vi "Construct.vi"(8 "error in (no error)":errorcluster, 11 "reference in":refnum<class "BrowerGuidencer.lvclass">) -> (0 "error out":errorcluster, 2 "BrowerComponent":refnum<class "BrowerComponent.lvclass">, 3 "reference out":refnum<class "BrowerGuidencer.lvclass">)   [LabVIEW 2015, in "BrowerGuidencer.lvclass"]
uses:
  BrowerGuidencer.lvclass
  BrowerComponent/BrowerComponent/BrowerComponent.lvclass
  BrowerGuidencer.lvclass/BrowerGuidencer.ctl
  AbstractBuilder/AbstractBuilder.lvclass
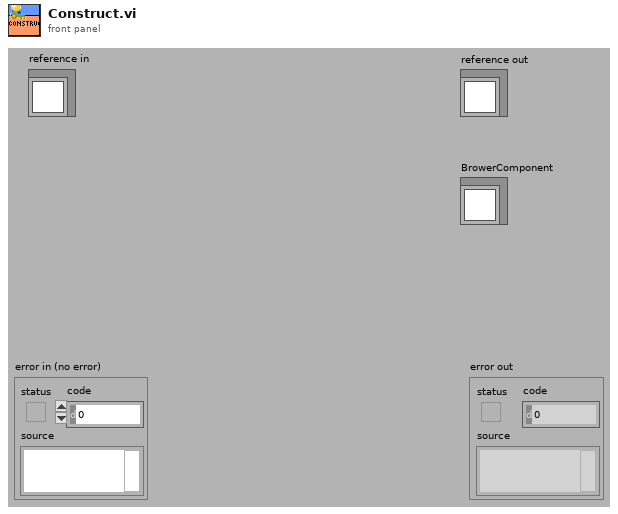
[diagram p1: front panel]
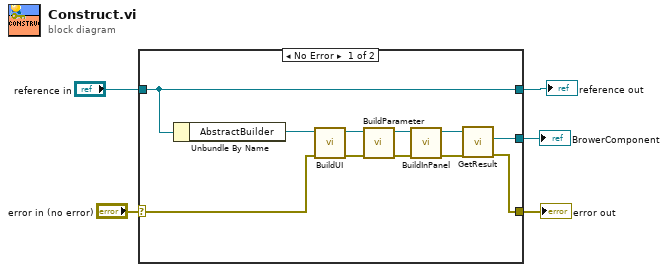
[diagram p0: block diagram]
diagram:
  n1 = case shown="No Error" "error in (no error)" {
    selector: "error in (no error)" -> [w14 w18]
    tunnel: [w7 w18] -> w4
    tunnel: [w16 w17] -> w2
    tunnel: "reference in" -> [w16 w17]
    tunnel: [w6 _] -> w1
    frame No Error {
      n2 = Unbundle By Name(w16) -> ("AbstractBuilder"=w15:refnum<class "AbstractBuilder.lvclass">)
      n3 = call-dynamic "BuildUI.vi"("error in (no error)"=w14, "reference in"=w15) -> ("error out"=w12:errorcluster, "reference out"=w13:refnum<class "AbstractBuilder.lvclass">)  [unwired: 8 in]
      n4 = call-dynamic "BuildParameter.vi"("error in (no error)"=w12, "AbstractBuilder in"=w13) -> ("error out"=w10:errorcluster, "AbstractBuilder out"=w11:refnum<class "AbstractBuilder.lvclass">)  [unwired: 8 in]
      n5 = call-dynamic "BuildInPanel.vi"("error in (no error)"=w10, "AbstractBuilder in"=w11) -> ("error out"=w8:errorcluster, "AbstractBuilder out"=w9:refnum<class "AbstractBuilder.lvclass">)  [unwired: 8 in]
      n6 = call-dynamic "GetResult.vi"("error in (no error)"=w8, "AbstractBuilder in"=w9) -> ("error out"=w7:errorcluster, "BrowerComponent"=w6:refnum<class "BrowerComponent.lvclass">)  [unwired: 7 in, 1 out]
    }
    frame Error {
    }
  }
  "error out" <- w4
  "reference out" <- w2
  "BrowerComponent" <- w1
